vi "Go To Starting Command.vi"(8 "error in (no error)":errorcluster, 11 "Command Processor in":refnum<class "Starting Command.lvclass">) -> (0 "error out":errorcluster, 3 "State out":refnum<class "State Actor.lvclass">)   [LabVIEW 2014, in "Robot Actor Framework.lvlib" / "Command Processor Actor.lvlib" / "Starting Command.lvclass"]
uses:
  Starting Command.lvclass
  <vilib>/ni/Actors/State Actor/State Actor/State Actor.lvclass
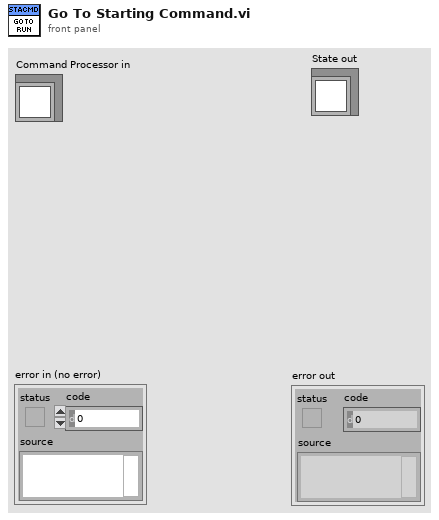
[diagram p1: front panel]
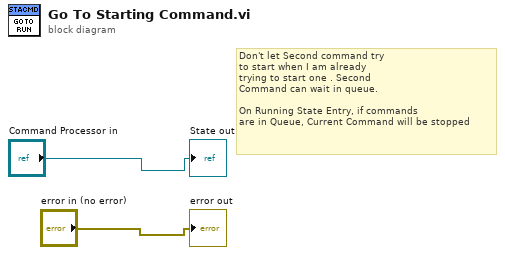
[diagram p0: block diagram]
diagram:
  # "Don't let Second command try \nto start when I am already\ntrying to start one . Second\nCommand can wait in queue.\n\nOn Running State Entry, if commands\nare in Queue, Current Command will be stopped"
  "error out" <- "error in (no error)"
  "State out" <- "Command Processor in"
